vi "specu1a 1.0.0 Close Pipe.vi"(3 "error in (no error)":errorcluster, 4 "Pipe Handle":i32, 5 "Device Handle":i32) -> (0 "error out":errorcluster, 2 "Device Handle out":i32)   [LabVIEW 2019]
uses:
  specu1a.dll
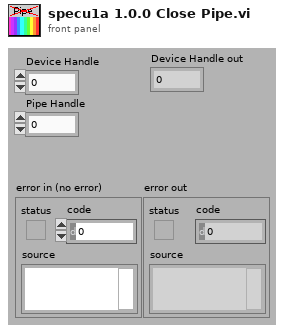
[diagram p1: front panel]
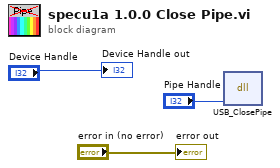
[diagram p0: block diagram]
diagram:
  n1 = dll-call lib="C:/Users/martzlab/Desktop/SIO 179/Nitrate/64/EvaluationSoftware/minispec labview/Hamamatsu Spectrometer Dll/specu1a.dll" fn="USB_ClosePipe" label="1.0.0 Close Pipe"("Pipe Handle"="Pipe Handle") -> ()  [unwired: 5 in, 2 out]
  "error out" <- "error in (no error)"
  "Device Handle out" <- "Device Handle"
